vi "Grdifruit Fridge Control program with improved reading and logging (1).vi"() -> ()   [LabVIEW 2020]
uses:
  03e38eda-cf4e-4072-9910-2f004f8baa0f.vi
  <extravilib>/ChannelInstances/Tag-dbl/Write With Abort.vi
  <extravilib>/ChannelInstances/Tag-exp/Write With Abort.vi
  <extravilib>/ChannelInstances/Tag-dbl/Read With Abort.vi
  <extravilib>/ChannelInstances/Tag-exp/Read With Abort.vi
  <extravilib>/ChannelInstances/Tag-bool/Write With Abort.vi
  <extravilib>/ChannelInstances/Tag-bool/Read With Abort.vi
  <extravilib>/ChannelInstances/Tag-c(stamp,stamp,stamp,a[.](dbl),dbl)/Read With Abort.vi
  <extravilib>/ChannelInstances/Tag-c(stamp,stamp,stamp,a[.](dbl),dbl)/Write With Abort.vi
  <extravilib>/ChannelInstances/Tag-c(stamp,stamp,stamp,a[.](dbl),dbl)/Instantiate.vi
  <extravilib>/ChannelInstances/Tag-c(stamp,stamp,stamp,a[.](dbl),dbl)/Endpoint.vi
  <extravilib>/ChannelInstances/Tag-dbl/Instantiate.vi
  <extravilib>/ChannelInstances/Tag-bool/Instantiate.vi
  <extravilib>/ChannelInstances/Tag-exp/Instantiate.vi
  <extravilib>/ChannelInstances/Tag-c(stamp,stamp,stamp,a[.](dbl),dbl)/EndpointRead.vi
  <extravilib>/ChannelInstances/Tag-dbl/EndpointRead.vi
  <extravilib>/ChannelInstances/Tag-bool/EndpointRead.vi
  <extravilib>/ChannelInstances/Tag-exp/EndpointRead.vi
  <vilib>/Analysis/2dsp.llb/Upsample (DBL).vi
  <vilib>/express/express shared/transition.llb/Dynamic To Waveform Array.vi
  <vilib>/express/express signal manip/GetorSetDDTAttributes/Set DDT Attributes/SetT0.vi
  <vilib>/express/express shared/transition.llb/Waveform Array To Dynamic.vi
  <extravilib>/ChannelInstances/Tag-dbl/Endpoint.vi
  <extravilib>/ChannelInstances/Tag-exp/Endpoint.vi
  <extravilib>/ChannelInstances/Tag-bool/Endpoint.vi
  <vilib>/express/express signal manip/GetorSetDDTAttributes/Set DDT Attributes/Set DDT Properties.xnode
  <extravilib>/ChannelInstances/Tag-bool.lvlib
  <extravilib>/ChannelInstances/Tag-dbl.lvlib
  <extravilib>/ChannelInstances/Tag-c(stamp,stamp,stamp,a[.](dbl),dbl).lvlib
  <extravilib>/ChannelInstances/Tag-exp.lvlib
  <vilib>/ptbypt/NI_PtbyPt.lvlib
  <vilib>/Analysis/NI_AALPro.lvlib
panel:
  out "Temperatures (present)":dbl[](array[numeric])
  out "Temperatures (historic)":dynamicdata(graph)
  out "Parsing error":string
  out "raw XML":string
  out "error out":errorcluster
  out "error out 2":errorcluster
  out "error out 3":errorcluster
  in  "Tab Control":T1(tab)
  in  "Minutes to start pre-cooling before event starts":dbl
  in  "Low temp boundary":dbl=15.0
  in  "High temp boundary":dbl=25.0
  in  "Desired Temp":dbl=20.0
  in  "Sample rate (Hz)":dbl=0.2
  in  "Samples":dbl=1.0
  in  "Timeout (Sec)":dbl=10.0
  in  "Enable Logging 2":bool caption="Enable"
  out "Saving/Logging Data 2":bool caption="Saving Data"
  in  "Path to log file 2":path=path "C:/Users/vwilso17/Documents/Grad School/testlogging.xlsx"
  in  "Append to Current File 2":bool caption="Enable"
  out "End time":timestamp
  out "Start time":timestamp
  in  "Poll ADR signal":bool
  out "Price":dbl
  out "duration":dbl[](array[numeric])
  in  "ADR file path":path=path "C:/Users/vwilso17/Documents/Grad School/projects/Grid Fruit HVAC Project/CPPpayload.txt"
  out "Current time":timestamp
  in  "Stop communication with PI":bool
  out "Temp Above Limit":bool
  out "Temp Below Limit":bool
  out "Compressor on":bool
  out "ADR enabled":bool
  in  "Short Cycle wait time (ms)":dbl
  in  "Enable Short cycle protection":bool
  # "Evaporator Surface\n\nInterior Air \n\nInterior Surface\n\nExterior surface"
  # "Timeout>=samples/sample rate\n\nor \n\nsample rate>=samples/Timeout"
  # "Weeks\nDays\nHour\nMinutes\nSeconds"
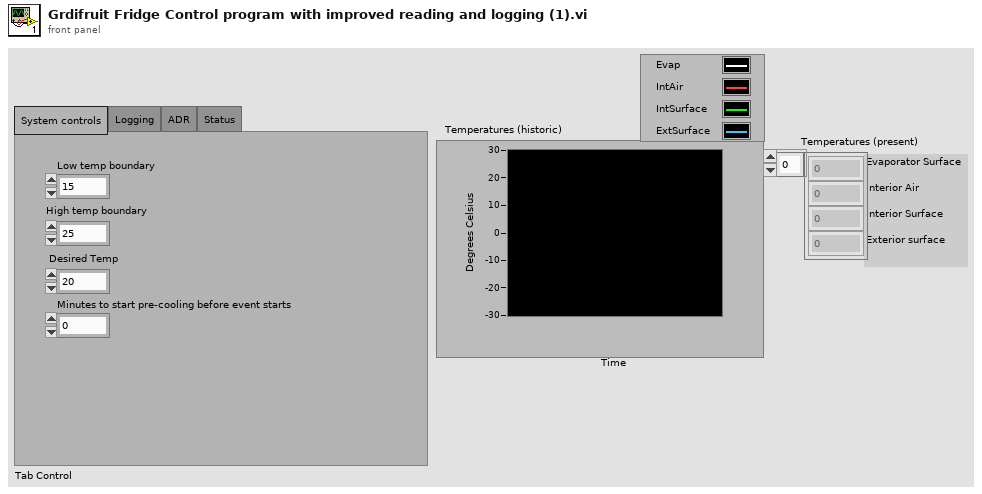
[diagram p1: front panel]
types:
  T1 = enum32{"System controls", "Logging", "ADR", "Status"}
  T2 = typedef "Tag-dbl.lvlib/))Channel.ctl" = refnum<queue>
  T3 = typedef "Tag-exp.lvlib/))Channel.ctl" = refnum<queue>
  T4 = cluster{"Current time":timestamp, "Start time":timestamp, "End time":timestamp, "duration":dbl[], "Price":dbl}
  T5 = cluster{"seconds since 1Jan1904":timestamp, "seconds since 1Jan1904":timestamp, "seconds since 1Jan1904":timestamp, "duration":dbl[], "Price":dbl}
  T6 = typedef "Tag-c(stamp,stamp,stamp,a[.](dbl),dbl).lvlib/))Channel.ctl" = refnum<queue>
  T7 = typedef "Tag-bool.lvlib/))Channel.ctl" = refnum<queue>
  T8 = enum16{"big-endian, network order", "native, host order", "little-endian"}
  T9 = cluster{"element":bool, "element":dbl, "element":dbl, "element":dbl, "element":dbl, "element":bool, timestamp, "Start time":timestamp, "End time":timestamp, "duration":dbl[], "Price":dbl, "element":dbl}
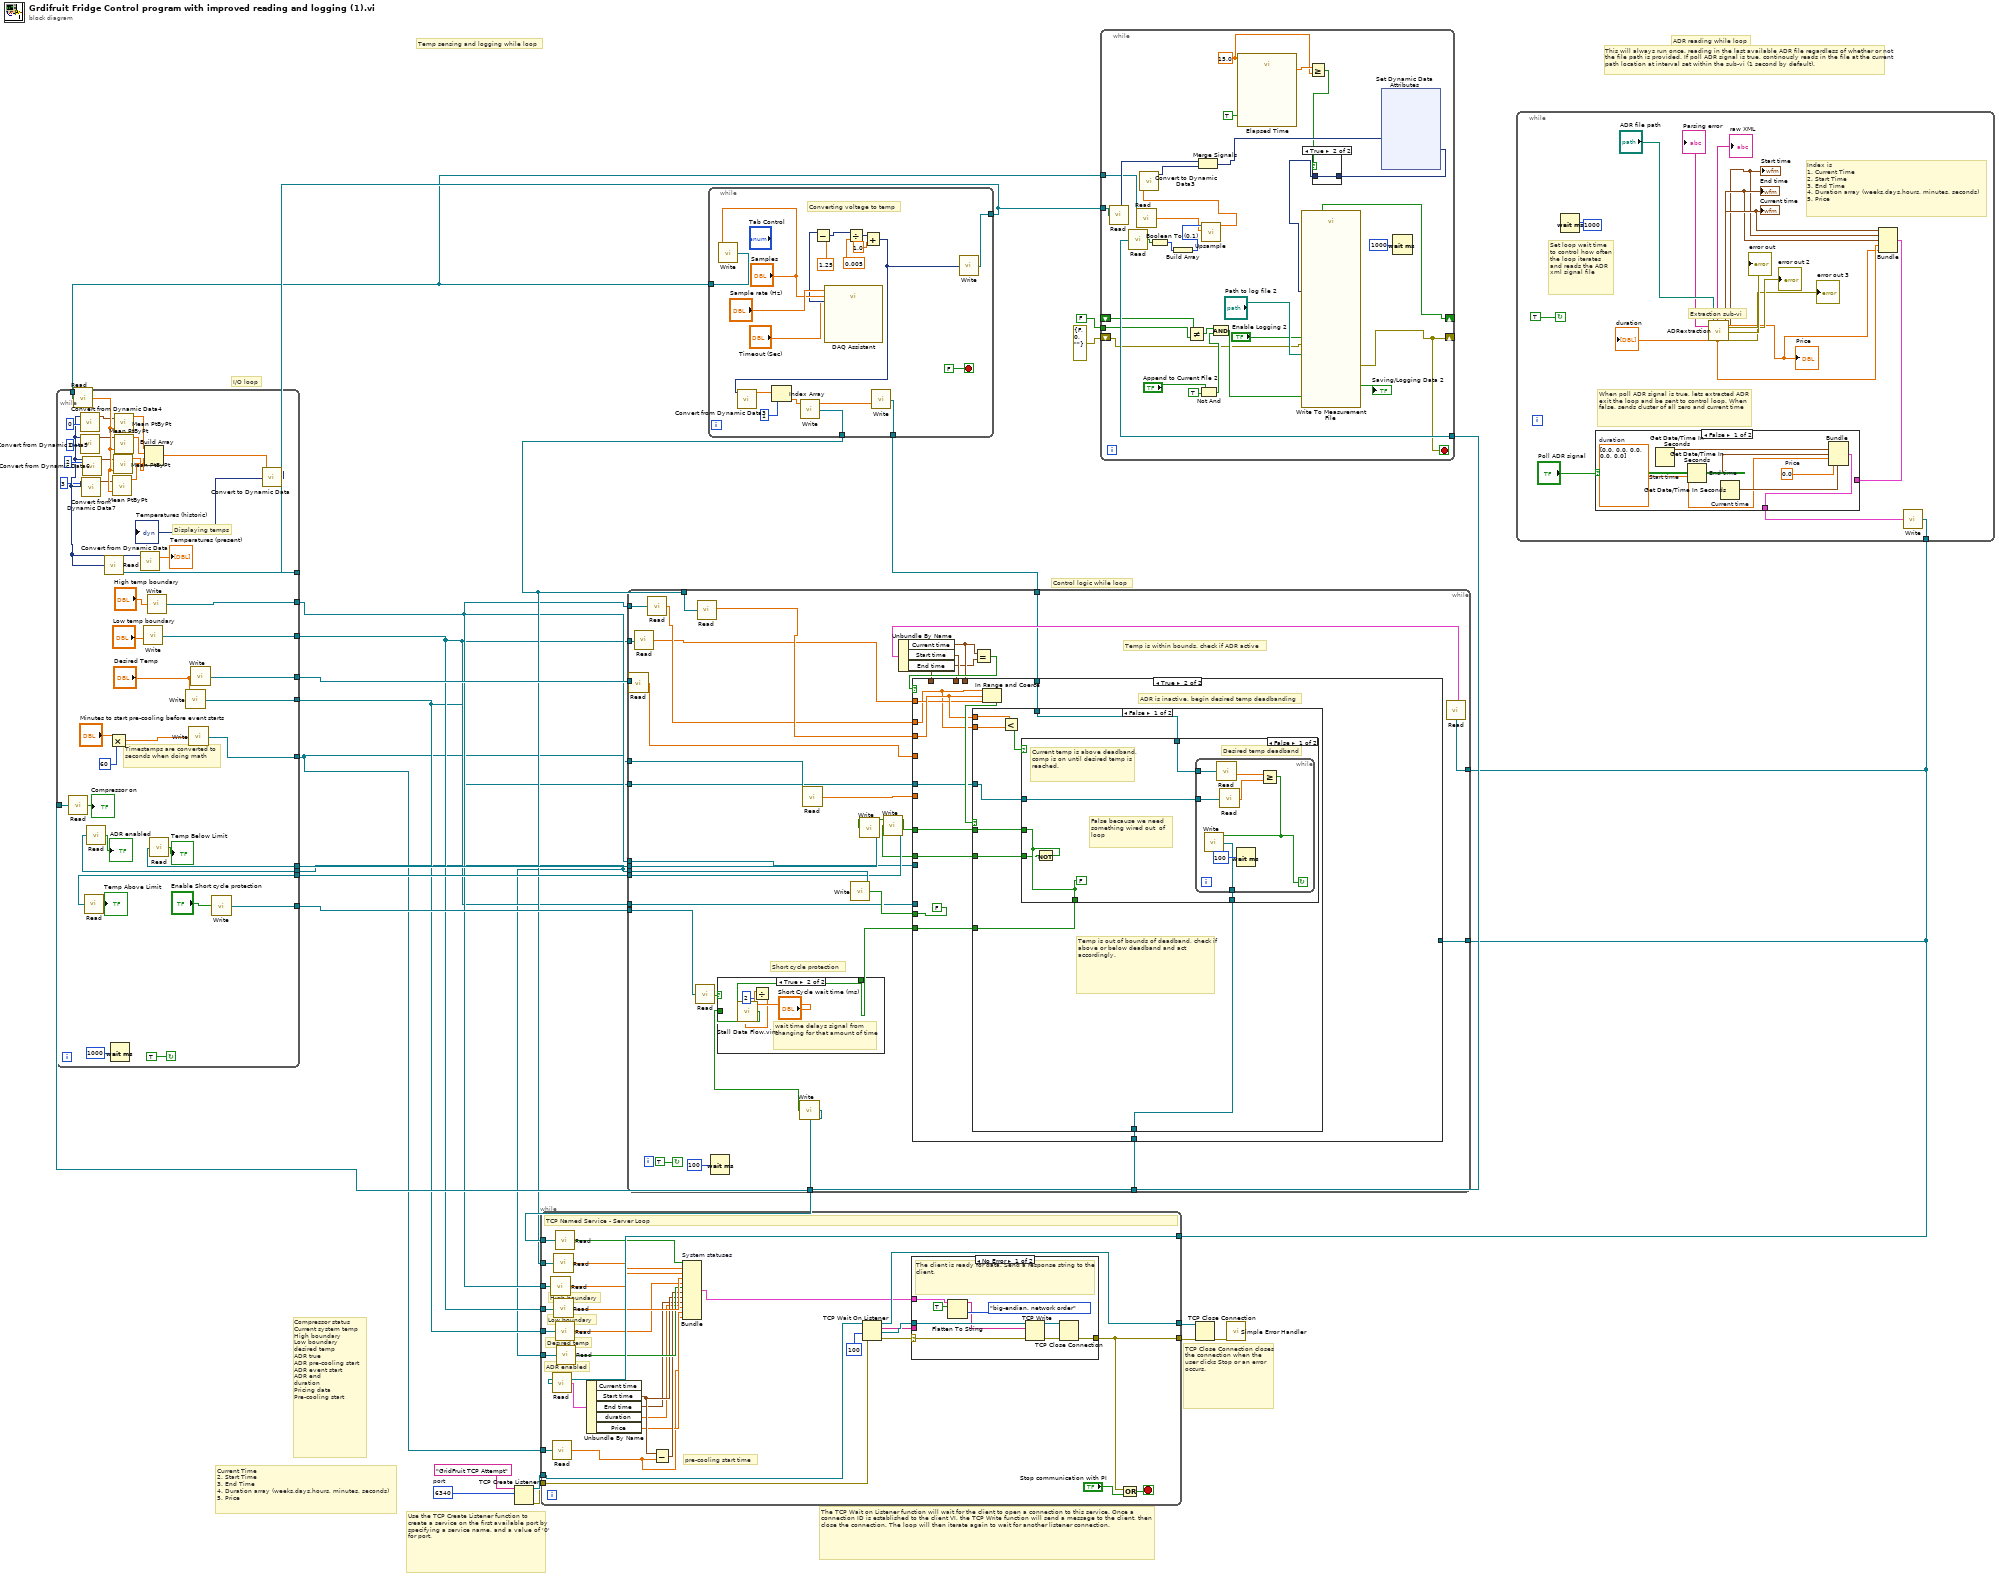
[diagram p0: block diagram]
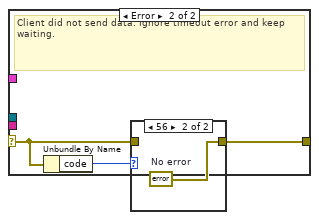
[diagram p3: hidden frame]
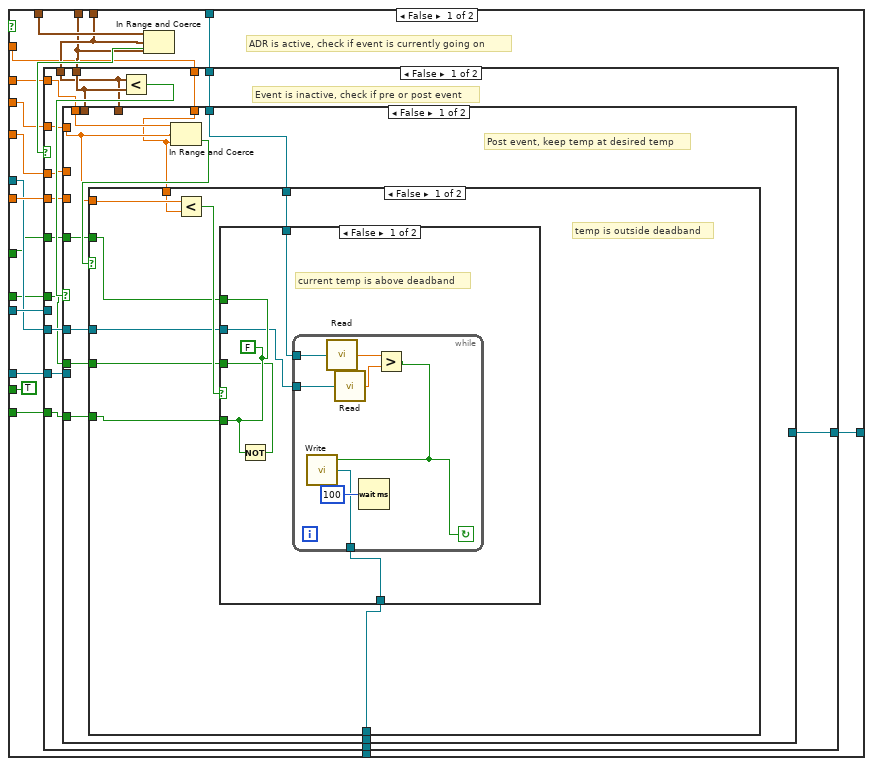
[diagram p5: hidden frame]
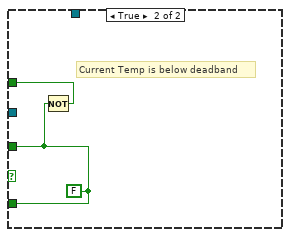
[diagram p6: hidden frame]
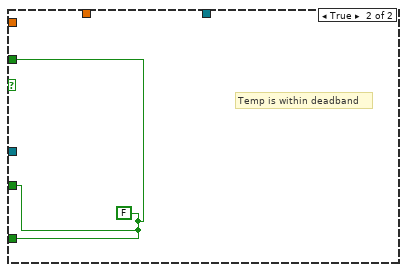
[diagram p7: hidden frame]
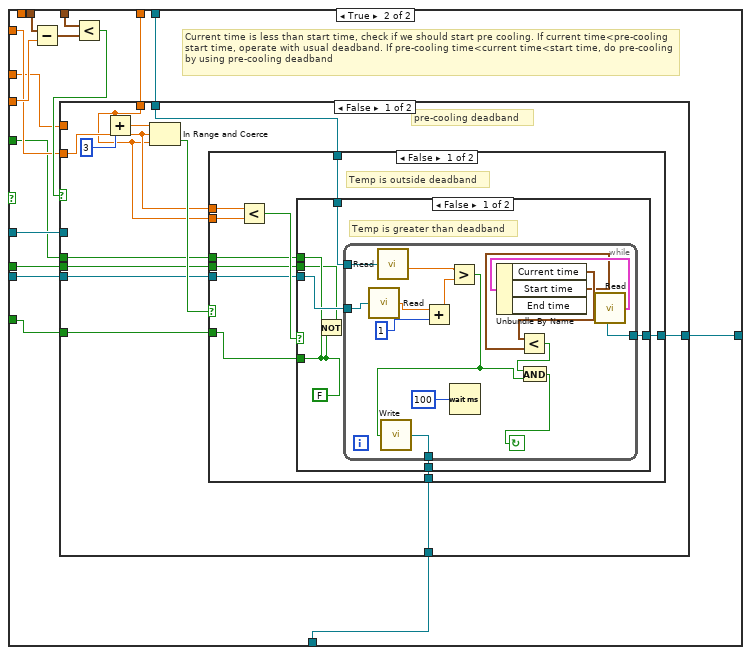
[diagram p8: hidden frame]
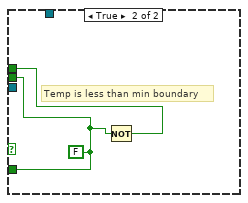
[diagram p9: hidden frame]
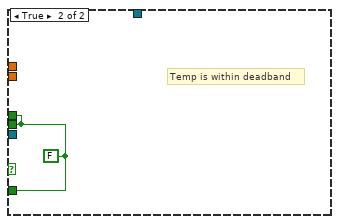
[diagram p10: hidden frame]
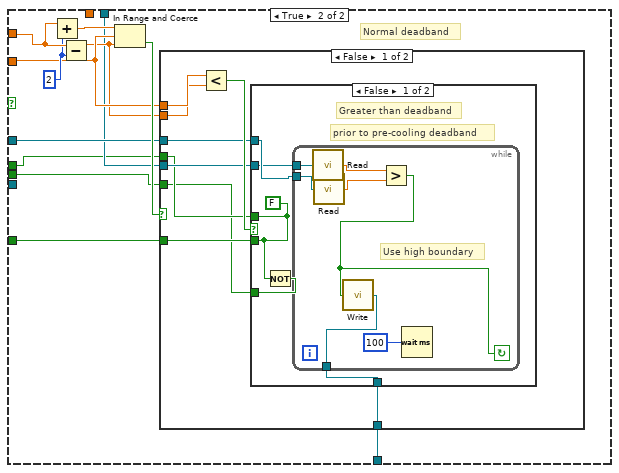
[diagram p11: hidden frame]
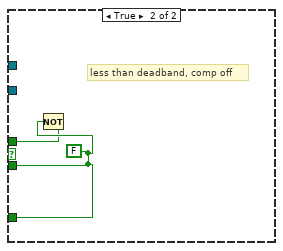
[diagram p12: hidden frame]
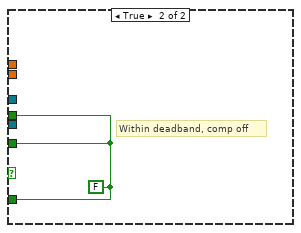
[diagram p13: hidden frame]
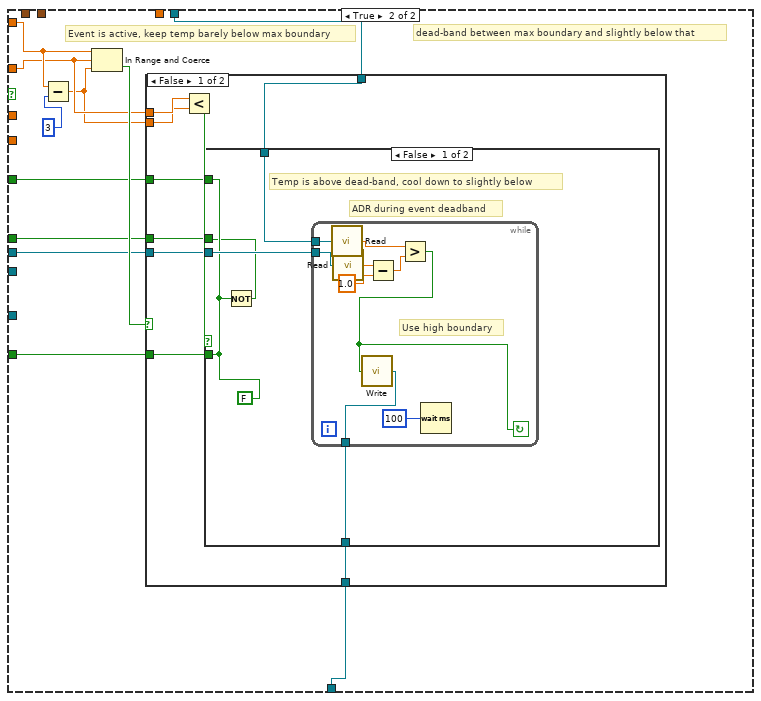
[diagram p14: hidden frame]
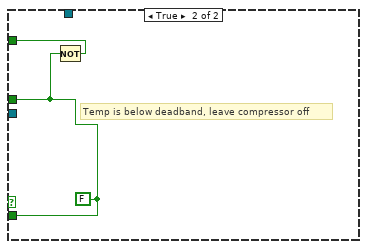
[diagram p15: hidden frame]
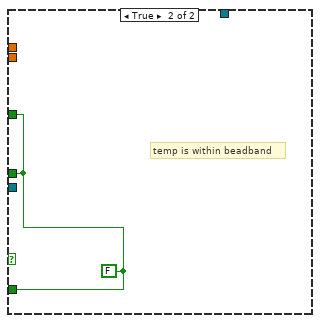
[diagram p16: hidden frame]
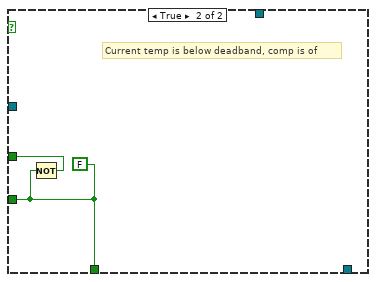
[diagram p17: hidden frame]
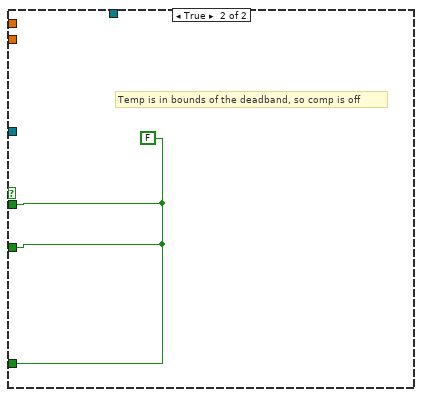
[diagram p18: hidden frame]
diagram:
  w19 = u16 6340  # port
  # "Current Time\n2. Start Time\n3. End Time\n4. Duration array (weeks,days,hours, minutes, seconds)\n5. Price"
  # "Compressor status\nCurrent system temp\nHigh boundary\nLow boundary\ndesired temp\nADR true\nADR pre-cooling start\nADR event start\nADR end\nduration\nPricing data\nPre-cooling start"
  # "I/O loop"
  # "TCP Close Connection closes the connection when the user clicks Stop or an error occurs."
  # "The TCP Wait on Listener function will wait for the client to open a connection to this service. Once a connection ID is established to the client VI, the TCP Write function will send a message to the client, then close the connection. The loop will then iterate again to wait for another listener connection."
  # "Use the TCP Create Listener function to create a service on the first available port by specifying a service name, and a value of '0' for port."
  # "Control logic while loop"
  # "Temp sensing and logging while loop"
  # "This will always run once, reading in the last available ADR file regardless of whether or not the file path is provided. If poll ADR signal is true, continously reads in the file at the current path location at interval set within the sub-vi (1 second by default)."
  # "ADR reading while loop"
  n1 = TCP Create Listener(10:w19, 11:"GridFruit TCP Attempt" ("service name")) -> (0:w23:errorcluster, 3:w24:refnum<k5>)  [unwired: 3 in, 1 out]
  n2 = while {
    tunnel: [w32] -> w7
    tunnel: [w31] -> w14
    tunnel: [w26] -> w9
    tunnel: [w25] -> w8
    stop <- FALSE stop-if-true
    # "Converting voltage to temp"
    n3 = call <extravilib>:"Write.vi"("element"="Samples") -> ("channel"=w25:T2)  [unwired: 1 out]
    n4 = call "DAQ Assistant"("rate"="Sample rate (Hz)", "number of samples"="Samples", "timeout (s)"="Timeout (Sec)") -> ("data"=w37:dynamicdata)  [unwired: 13 in, 3 out]
    n5 = Subtract(x=w37, y=1.25) -> (x-y=w40:dynamicdata)
    n6 = Divide(x=w40, y=0.005) -> (x/y=w30:dynamicdata)
    n7 = Add(x=w30, y=1.0) -> (x+y=w27:dynamicdata)
    n8 = call "Convert from Dynamic Data3"("Dynamic Data Type"=w27) -> ("Array"=w35:dbl[])  [unwired: 3 in]
    n9 = Index Array(array=w35, index=1) -> (element=w33:dbl)
    n10 = call <extravilib>:"Write.vi"("element"=w33) -> ("channel"=w32:T2)  [unwired: 1 out]
    n11 = call <extravilib>:"Write.vi"("element"=w33) -> ("channel"=w31:T2)  [unwired: 1 out]
    n12 = call <extravilib>:"Write.vi"("element"=w27) -> ("channel"=w26:T3)  [unwired: 1 out]
  }
  n13 = while {
    tunnel: [w44] -> w1
    stop <- TRUE continue-if-true
    # "Index is\n1. Current Time\n2. Start Time\n3. End Time\n4. Duration array (weeks,days,hours, minutes, seconds)\n5. Price"
    # "Set loop wait time to control how often the loop iterates and reads the ADR xml signal file"
    # "When poll ADR signal is true, lets extracted ADR exit the loop and be sent to control loop. When false, sends cluster of all zero and current time"
    # "Extraction sub-vi"
    n14 = Wait (ms)(milliseconds to wait=1000) -> ()  [unwired: 1 out]
    n15 = call "ADRextraction.vi"("Path in"="ADR file path") -> ("Error"=→"Parsing error":string, "raw xML"=→"raw XML":string, "duration"=w46:dbl[], "Start time"=w43:timestamp, "End time"=w51:timestamp, "Current time"=w52:timestamp, "Price"=w45:dbl, "error out 2"=→"error out 2":errorcluster, 24:"error out"=→"error out":errorcluster, 27:"error out"=→"error out 3":errorcluster)  [unwired: 12 in, 5 out]
    "Price" <- w45
    "duration" <- w46
    "Start time" <- w43
    "End time" <- w51
    "Current time" <- w52
    n16 = Bundle("Current time"=w52, "Start time"=w43, "End time"=w51, "duration"=w46, "Price"=w45) -> (w47:T4)  [unwired: 1 in]
    n17 = case shown="False" "Poll ADR signal" {
      tunnel: [w61 w66] -> w48
      tunnel: w47 -> [_ w66]
      frame False {
        w60 = dbl[] [0.0, 0.0, 0.0, 0.0, 0.0]  # duration
        w62 = 0.0  # Price
        n18 = Get Date/Time In Seconds "Start time"() -> (seconds since 1Jan1904=w63:timestamp)
        n19 = Get Date/Time In Seconds "End time"() -> (seconds since 1Jan1904=w64:timestamp)
        n20 = Get Date/Time In Seconds "Current time"() -> (seconds since 1Jan1904=w65:timestamp)
        n21 = Bundle("seconds since 1Jan1904"=w65, "seconds since 1Jan1904"=w63, "seconds since 1Jan1904"=w64, "duration"=w60, "Price"=w62) -> (w61:T5)  [unwired: 1 in]
      }
      frame True {
      }
    }
    n22 = call <extravilib>:"Write.vi"("element"=w48) -> ("channel"=w44:T6)  [unwired: 1 out]
  }
  n23 = while {
    tunnel: [w106] -> w6
    tunnel: [w104] -> w5
    tunnel: [w102] -> w18
    tunnel: [w98] -> w2
    tunnel: w12 -> [w96]
    tunnel: w3 -> [w94]
    tunnel: w17 -> [w92]
    tunnel: w16 -> [w90]
    tunnel: [w87] -> w15
    tunnel: [w86] -> w4
    tunnel: w9 -> [w85]
    tunnel: w8 -> [w81]
    stop <- TRUE continue-if-true
    # "Displaying temps"
    # "Timestamps are converted to seconds when doing math"
    n24 = call <extravilib>:"Read.vi"("channel"=w96) -> ("element"=→"Compressor on":bool)  [unwired: 1 in, 1 out]
    n25 = call <extravilib>:"Read.vi"("channel"=w81) -> ("element"=w77:dbl)  [unwired: 1 in, 1 out]
    n26 = call <extravilib>:"Read.vi"("channel"=w90) -> ("element"=→"Temp Above Limit":bool)  [unwired: 1 in, 1 out]
    n27 = call <extravilib>:"Read.vi"("channel"=w94) -> ("element"=→"ADR enabled":bool)  [unwired: 1 in, 1 out]
    n28 = call <extravilib>:"Read.vi"("channel"=w85) -> ("element"=w71:dynamicdata)  [unwired: 1 in, 1 out]
    n29 = call "Convert from Dynamic Data4"("Dynamic Data Type"=w71, "Channel"=0) -> ("Waveform"=w76:waveform(dbl))  [unwired: 2 in]
    n30 = call "Convert from Dynamic Data5"("Dynamic Data Type"=w71, "Channel"=1) -> ("Waveform"=w75:waveform(dbl))  [unwired: 2 in]
    n31 = call "Convert from Dynamic Data7"("Dynamic Data Type"=w71, "Channel"=3) -> ("Waveform"=w70:waveform(dbl))  [unwired: 2 in]
    n32 = call "Convert from Dynamic Data6"("Dynamic Data Type"=w71, "Channel"=2) -> ("Waveform"=w73:waveform(dbl))  [unwired: 2 in]
    n33 = Multiply(x="Minutes to start pre-cooling before event starts", y=60) -> (x*y=w99:dbl)
    n34 = Wait (ms)(milliseconds to wait=u32 1000) -> ()  [unwired: 1 out]
    n35 = call <vilib>:"Mean PtByPt.vi"("x"=w70, "sample length"=w77) -> ("mean"=w78:dbl)  [unwired: 2 in, 1 out]
    n36 = call <vilib>:"Mean PtByPt.vi"("x"=w73, "sample length"=w77) -> ("mean"=w79:dbl)  [unwired: 2 in, 1 out]
    n37 = call <vilib>:"Mean PtByPt.vi"("x"=w76, "sample length"=w77) -> ("mean"=w84:dbl)  [unwired: 2 in, 1 out]
    n38 = call <vilib>:"Mean PtByPt.vi"("x"=w75, "sample length"=w77) -> ("mean"=w80:dbl)  [unwired: 2 in, 1 out]
    n39 = call "Convert from Dynamic Data"("Dynamic Data Type"=w71) -> ("Array"=→"Temperatures (present)":dbl[])  [unwired: 3 in]
    n40 = call <extravilib>:"Write.vi"("element"="Low temp boundary") -> ("channel"=w104:T2)  [unwired: 1 out]
    n41 = Build Array(w84, w80, w79, w78) -> (w83:dbl[])
    n42 = call <extravilib>:"Write.vi"("element"="High temp boundary") -> ("channel"=w106:T2)  [unwired: 1 out]
    n43 = call <extravilib>:"Read.vi"("channel"=w92) -> ("element"=→"Temp Below Limit":bool)  [unwired: 1 in, 1 out]
    n44 = call <extravilib>:"Write.vi"("element"="Desired Temp") -> ("channel"=w86:T2)  [unwired: 1 out]
    n45 = call <extravilib>:"Write.vi"("element"=w99) -> ("channel"=w98:T2)  [unwired: 1 out]
    n46 = call <extravilib>:"Write.vi"("element"="Desired Temp") -> ("channel"=w102:T2)  [unwired: 1 out]
    n47 = call <extravilib>:"Write.vi"("element"="Enable Short cycle protection") -> ("channel"=w87:T7)  [unwired: 1 out]
    n48 = call "Convert to Dynamic Data"("Array"=w83) -> ("Dynamic Data Type"=→"Temperatures (historic)":dynamicdata)  [unwired: 3 in]
  }
  n49 = while {
    tunnel: w1 -> [w140]
    tunnel: w7 -> [w137]
    tunnel: w6 -> [w135]
    tunnel: w5 -> [w133]
    tunnel: w18 -> [w131]
    tunnel: w2 -> [w129]
    tunnel: [w127] -> w12
    tunnel: [w125] -> w3
    tunnel: [w124] -> w17
    tunnel: [w123] -> w16
    tunnel: w15 -> [w122]
    tunnel: w4 -> [w120]
    tunnel: w14 -> [w119]
    tunnel: w12 -> [w118]
    tunnel: w6 -> [w117]
    tunnel: w5 -> [w116]
    tunnel: w1 -> [w109]
    stop <- TRUE continue-if-true
    # "Temp is within bounds, check if ADR active"
    # "Short cycle protection"
    n50 = call <extravilib>:"Read.vi"("channel"=w131) -> ("element"=w130:dbl)  [unwired: 1 in, 1 out]
    n51 = call <extravilib>:"Read.vi"("channel"=w133) -> ("element"=w132:dbl)  [unwired: 1 in, 1 out]
    n52 = call <extravilib>:"Read.vi"("channel"=w135) -> ("element"=w134:dbl)  [unwired: 1 in, 1 out]
    n53 = call <extravilib>:"Read.vi"("channel"=w122) -> ("element"=w121:bool)  [unwired: 1 in, 1 out]
    n54 = call <extravilib>:"Read.vi"("channel"=w137) -> ("element"=w136:dbl)  [unwired: 1 in, 1 out]
    n55 = Wait (ms)(milliseconds to wait=u32 100) -> ()  [unwired: 1 out]
    n56 = call <extravilib>:"Read.vi"("channel"=w129) -> ("element"=w128:dbl)  [unwired: 1 in, 1 out]
    n57 = call <extravilib>:"Read.vi"("channel"=w140) -> ("element"=w139:T4)  [unwired: 1 in, 1 out]
    n58 = Unbundle By Name(w139) -> ("Current time"=w114:timestamp, "Start time"=w113:timestamp, "End time"=w112:timestamp)
    n59 = Equal?(x=w114, y=w112) -> (x = y?=w115:bool)
    n60 = case shown="True" w115 {
      tunnel: w136 -> [w157 w355]
      tunnel: w130 -> [w156 _]
      tunnel: [w155 w357] -> w143
      tunnel: [TRUE FALSE] -> w126
      tunnel: w114 -> [w159 _]
      tunnel: w113 -> [w158 _]
      tunnel: w112 -> [w161 _]
      tunnel: w134 -> [w154 w348]
      tunnel: w128 -> [w153 _]
      tunnel: w132 -> [w152 w349]
      tunnel: w120 -> [w147 w354]
      tunnel: w119 -> [w150 w353]
      tunnel: [w149 w352] -> w118
      tunnel: w117 -> [w151 _]
      tunnel: w116 -> [w148 _]
      tunnel: [w146 w351] -> w111
      tunnel: [w145 w350] -> w110
      tunnel: w109 -> [w144 _]
      frame False {
        # "ADR is active, check if event is currently going on"
        n61 = In Range and Coerce(upper limit=w161, x=w159, lower limit=w158) -> (In Range?=w160:bool)  [unwired: 1 out]
        n62 = case shown="False" w160 {
          tunnel: w159 -> [w172 _]
          tunnel: w158 -> [w173 _]
          tunnel: w157 -> [w177 w317]
          tunnel: w156 -> [w176 _]
          tunnel: [w175 w318] -> w155
          tunnel: w154 -> [w163 w321]
          tunnel: w153 -> [w174 _]
          tunnel: w152 -> [w171 _]
          tunnel: w151 -> [_ w315]
          tunnel: w150 -> [w170 w314]
          tunnel: [w169 w313] -> w149
          tunnel: w148 -> [w168 _]
          tunnel: w147 -> [w167 _]
          tunnel: [w166 w312] -> w146
          tunnel: [w165 w311] -> w145
          tunnel: w144 -> [w164 _]
          frame False {
            # "Event is inactive, check if pre or post event"
            n63 = Less?(x=w172, y=w173) -> (x < y?=w178:bool)
            n64 = case shown="False" w178 {
              tunnel: w177 -> [w186 w223]
              tunnel: w176 -> [_ w222]
              tunnel: [w187 w221] -> w175
              tunnel: w174 -> [_ w228]
              tunnel: w173 -> [_ w227]
              tunnel: w172 -> [_ w226]
              tunnel: w171 -> [w180 w220]
              tunnel: w170 -> [w185 w218]
              tunnel: [w184 w219] -> w169
              tunnel: w168 -> [_ w217]
              tunnel: w167 -> [w179 w216]
              tunnel: [w183 w215] -> w166
              tunnel: [w182 w214] -> w165
              tunnel: w164 -> [_ w213]
              tunnel: w163 -> [w181 _]
              frame False {
                # "Post event, keep temp at desired temp"
                n65 = In Range and Coerce(upper limit=w181, x=w186, lower limit=w180) -> (In Range?=w188:bool)  [unwired: 1 out]
                n66 = case shown="False" w188 {
                  tunnel: [w195 w212] -> w187
                  tunnel: w186 -> [w197 _]
                  tunnel: w185 -> [w194 _]
                  tunnel: [w193 _] -> w184
                  tunnel: [w192 w212] -> w183
                  tunnel: [w191 w212] -> w182
                  tunnel: w180 -> [w190 _]
                  tunnel: w179 -> [w189 _]
                  frame False {
                    # "temp is outside deadband"
                    n67 = Less?(x=w197, y=w190) -> (x < y?=w196:bool)
                    n68 = case shown="False" w196 {
                      tunnel: [w200 w211] -> w195
                      tunnel: w194 -> [w202 _]
                      tunnel: [w201 _] -> w193
                      tunnel: [w199 w211] -> w192
                      tunnel: [w200 w210] -> w191
                      tunnel: w189 -> [w198 _]
                      frame False {
                        w200 = FALSE
                        # "current temp is above deadband"
                        n69 = Not(x=w200) -> (.not. x?=w199:bool)
                        n70 = while {
                          tunnel: w202 -> [w208]
                          tunnel: [w207] -> w201
                          tunnel: w198 -> [w204]
                          stop <- w205 continue-if-true
                          n71 = call <extravilib>:"Read.vi"("channel"=w208) -> ("element"=w206:dbl)  [unwired: 1 in, 1 out]
                          n72 = call <extravilib>:"Read.vi"("channel"=w204) -> ("element"=w203:dbl)  [unwired: 1 in, 1 out]
                          n73 = Wait (ms)(milliseconds to wait=u32 100) -> ()  [unwired: 1 out]
                          n74 = Greater?(x=w206, y=w203) -> (0:w205:bool)
                          n75 = call <extravilib>:"Write.vi"("element"=w205) -> ("channel"=w207:T7)  [unwired: 1 out]
                        }
                      }
                      frame True {
                        w211 = FALSE
                        # "Current Temp is below deadband"
                        n76 = Not(x=w211) -> (.not. x?=w210:bool)
                      }
                    }
                  }
                  frame True {
                    w212 = FALSE
                    # "Temp is within deadband"
                  }
                }
              }
              frame True {
                # "Current time is less than start time, check if we should start pre cooling. If current time<pre-cooling start time, operate with usual deadband. If pre-cooling time<current time<start time, do pre-cooling by using pre-cooling deadband"
                n77 = Subtract(x=w227, y=w228) -> (x-y=w225:timestamp)
                n78 = Less?(x=w226, y=w225) -> (x < y?=w224:bool)
                n79 = case shown="False" w224 {
                  tunnel: w223 -> [w237 w281]
                  tunnel: w222 -> [_ w285]
                  tunnel: [w235 w282] -> w221
                  tunnel: w220 -> [w236 _]
                  tunnel: [w234 w277] -> w219
                  tunnel: w218 -> [w233 w278]
                  tunnel: w217 -> [w232 _]
                  tunnel: w216 -> [_ w279]
                  tunnel: [w231 w276] -> w215
                  tunnel: [w230 w275] -> w214
                  tunnel: w213 -> [w229 _]
                  frame False {
                    # "pre-cooling deadband"
                    n80 = Add(x=w236, y=3) -> (x+y=w239:dbl)
                    n81 = In Range and Coerce(upper limit=w239, x=w237, lower limit=w236) -> (In Range?=w238:bool)  [unwired: 1 out]
                    n82 = case shown="False" w238 {
                      tunnel: w237 -> [w248 _]
                      tunnel: w236 -> [w247 _]
                      tunnel: [w249 w274] -> w235
                      tunnel: [w246 _] -> w234
                      tunnel: w233 -> [w245 _]
                      tunnel: w232 -> [w244 _]
                      tunnel: [w242 w274] -> w231
                      tunnel: [w243 w274] -> w230
                      tunnel: w229 -> [w241 _]
                      frame False {
                        # "Temp is outside deadband"
                        n83 = Less?(x=w248, y=w247) -> (x < y?=w250:bool)
                        n84 = case shown="False" w250 {
                          tunnel: [w253 w273] -> w249
                          tunnel: [w256 _] -> w246
                          tunnel: w245 -> [w255 _]
                          tunnel: w244 -> [w254 _]
                          tunnel: [w253 w272] -> w243
                          tunnel: [w252 w273] -> w242
                          tunnel: w241 -> [w251 _]
                          frame False {
                            w253 = FALSE
                            # "Temp is greater than deadband"
                            n85 = Not(x=w253) -> (.not. x?=w252:bool)
                            n86 = while {
                              tunnel: w254 -> [w270]
                              tunnel: w255 -> [w269]
                              tunnel: [w268] -> w256
                              tunnel: w251 -> [w263]
                              stop <- w261 continue-if-true
                              n87 = call <extravilib>:"Read.vi"("channel"=w270) -> ("element"=w266:dbl)  [unwired: 1 in, 1 out]
                              n88 = call <extravilib>:"Read.vi"("channel"=w269) -> ("element"=w264:dbl)  [unwired: 1 in, 1 out]
                              n89 = Add(x=w266, y=1) -> (x+y=w265:dbl)
                              n90 = Greater?(x=w264, y=w265) -> (0:w260:bool)
                              n91 = call <extravilib>:"Write.vi"("element"=w260) -> ("channel"=w268:T7)  [unwired: 1 out]
                              n92 = Wait (ms)(milliseconds to wait=u32 100) -> ()  [unwired: 1 out]
                              n93 = call <extravilib>:"Read.vi"("channel"=w263) -> ("element"=w262:T4)  [unwired: 1 in, 1 out]
                              n94 = Unbundle By Name(w262) -> ("Current time"=w259:timestamp, "Start time"=w258:timestamp)  [unwired: 1 out]
                              n95 = Less?(x=w259, y=w258) -> (x < y?=w257:bool)
                              n96 = And(x=w257, y=w260) -> (x .and. y?=w261:bool)
                            }
                          }
                          frame True {
                            w273 = FALSE
                            # "Temp is less than min boundary"
                            n97 = Not(x=w273) -> (.not. x?=w272:bool)
                          }
                        }
                      }
                      frame True {
                        w274 = FALSE
                        # "Temp is within deadband"
                      }
                    }
                  }
                  frame True {
                    w284 = 2
                    # "Normal deadband"
                    n98 = Add(x=w285, y=w284) -> (x+y=w286:dbl)
                    n99 = Subtract(x=w285, y=w284) -> (x-y=w280:dbl)
                    n100 = In Range and Coerce(upper limit=w286, x=w281, lower limit=w280) -> (In Range?=w283:bool)  [unwired: 1 out]
                    n101 = case shown="False" w283 {
                      tunnel: [w292 w310] -> w282
                      tunnel: w281 -> [w295 _]
                      tunnel: w280 -> [w294 _]
                      tunnel: w279 -> [w291 _]
                      tunnel: w278 -> [w290 _]
                      tunnel: [w289 _] -> w277
                      tunnel: [w287 w310] -> w276
                      tunnel: [w288 w310] -> w275
                      frame False {
                        n102 = Less?(x=w295, y=w294) -> (x < y?=w293:bool)
                        n103 = case shown="False" w293 {
                          tunnel: [w297 w309] -> w292
                          tunnel: w291 -> [w300 _]
                          tunnel: w290 -> [w299 _]
                          tunnel: [w298 _] -> w289
                          tunnel: [w297 w308] -> w288
                          tunnel: [w296 w309] -> w287
                          frame False {
                            w297 = FALSE
                            # "prior to pre-cooling deadband"
                            # "Greater than deadband"
                            n104 = Not(x=w297) -> (.not. x?=w296:bool)
                            n105 = while {
                              tunnel: [w305] -> w298
                              tunnel: w300 -> [w303]
                              tunnel: w299 -> [w302]
                              stop <- w304 continue-if-true
                              # "Use high boundary"
                              n106 = call <extravilib>:"Read.vi"("channel"=w302) -> ("element"=w306:dbl)  [unwired: 1 in, 1 out]
                              n107 = call <extravilib>:"Read.vi"("channel"=w303) -> ("element"=w301:dbl)  [unwired: 1 in, 1 out]
                              n108 = Greater?(x=w306, y=w301) -> (0:w304:bool)
                              n109 = call <extravilib>:"Write.vi"("element"=w304) -> ("channel"=w305:T7)  [unwired: 1 out]
                              n110 = Wait (ms)(milliseconds to wait=u32 100) -> ()  [unwired: 1 out]
                            }
                          }
                          frame True {
                            w309 = FALSE
                            # "less than deadband, comp off"
                            n111 = Not(x=w309) -> (.not. x?=w308:bool)
                          }
                        }
                      }
                      frame True {
                        w310 = FALSE
                        # "Within deadband, comp off"
                      }
                    }
                  }
                }
              }
            }
          }
          frame True {
            # "dead-band between max boundary and slightly below that"
            # "Event is active, keep temp barely below max boundary"
            n112 = Subtract(x=w321, y=3) -> (x-y=w316:dbl)
            n113 = In Range and Coerce(upper limit=w321, x=w317, lower limit=w316) -> (In Range?=w319:bool)  [unwired: 1 out]
            n114 = case shown="False" w319 {
              tunnel: [w327 w347] -> w318
              tunnel: w317 -> [w330 _]
              tunnel: w316 -> [w329 _]
              tunnel: [w326 _] -> w313
              tunnel: w315 -> [w325 _]
              tunnel: w314 -> [w324 _]
              tunnel: [w323 w347] -> w312
              tunnel: [w322 w347] -> w311
              frame False {
                n115 = Less?(x=w330, y=w329) -> (x < y?=w328:bool)
                n116 = case shown="False" w328 {
                  tunnel: [w332 w346] -> w327
                  tunnel: [w335 _] -> w326
                  tunnel: w325 -> [w334 _]
                  tunnel: w324 -> [w333 _]
                  tunnel: [w331 w346] -> w323
                  tunnel: [w332 w345] -> w322
                  frame False {
                    w332 = FALSE
                    # "ADR during event deadband"
                    # "Temp is above dead-band, cool down to slightly below"
                    n117 = Not(x=w332) -> (.not. x?=w331:bool)
                    n118 = while {
                      tunnel: [w339] -> w335
                      tunnel: w334 -> [w337]
                      tunnel: w333 -> [w336]
                      stop <- w338 continue-if-true
                      # "Use high boundary"
                      n119 = call <extravilib>:"Read.vi"("channel"=w336) -> ("element"=w341:dbl)  [unwired: 1 in, 1 out]
                      n120 = call <extravilib>:"Read.vi"("channel"=w337) -> ("element"=w343:dbl)  [unwired: 1 in, 1 out]
                      n121 = Subtract(x=w343, y=1.0) -> (x-y=w340:dbl)
                      n122 = Greater?(x=w341, y=w340) -> (0:w338:bool)
                      n123 = call <extravilib>:"Write.vi"("element"=w338) -> ("channel"=w339:T7)  [unwired: 1 out]
                      n124 = Wait (ms)(milliseconds to wait=u32 100) -> ()  [unwired: 1 out]
                    }
                  }
                  frame True {
                    w346 = FALSE
                    # "Temp is below deadband, leave compressor off"
                    n125 = Not(x=w346) -> (.not. x?=w345:bool)
                  }
                }
              }
              frame True {
                w347 = FALSE
                # "temp is within beadband"
              }
            }
          }
        }
      }
      frame True {
        # "ADR is inactive, begin desired temp deadbanding"
        n126 = In Range and Coerce(upper limit=w348, x=w355, lower limit=w349) -> (In Range?=w358:bool)  [unwired: 1 out]
        n127 = case shown="False" w358 {
          tunnel: [w365 w382] -> w357
          tunnel: w355 -> [w367 _]
          tunnel: w354 -> [w364 _]
          tunnel: w353 -> [w363 _]
          tunnel: [w362 _] -> w352
          tunnel: [w361 w382] -> w351
          tunnel: [w360 w382] -> w350
          tunnel: w348 -> [w359 _]
          frame False {
            # "Temp is out of bounds of deadband, check if above or below deadband and act accordingly."
            n128 = Less?(x=w367, y=w359) -> (x < y?=w366:bool)
            n129 = case shown="False" w366 {
              tunnel: [w369 w381] -> w365
              tunnel: w364 -> [w372 _]
              tunnel: w363 -> [w371 _]
              tunnel: [w370 _] -> w362
              tunnel: [w368 w381] -> w361
              tunnel: [w369 w380] -> w360
              frame False {
                w369 = FALSE
                # "Desired temp deadband"
                # "False because we need something wired out  of loop"
                # "Current temp is above deadband, comp is on until desired temp is reached."
                n130 = Not(x=w369) -> (.not. x?=w368:bool)
                n131 = while {
                  tunnel: w372 -> [w377]
                  tunnel: w371 -> [w375]
                  tunnel: [w374] -> w370
                  stop <- w373 continue-if-true
                  n132 = call <extravilib>:"Read.vi"("channel"=w375) -> ("element"=w378:dbl)  [unwired: 1 in, 1 out]
                  n133 = call <extravilib>:"Read.vi"("channel"=w377) -> ("element"=w376:dbl)  [unwired: 1 in, 1 out]
                  n134 = Wait (ms)(milliseconds to wait=u32 100) -> ()  [unwired: 1 out]
                  n135 = Greater Or Equal?(x=w378, y=w376) -> (x >= y?=w373:bool)
                  n136 = call <extravilib>:"Write.vi"("element"=w373) -> ("channel"=w374:T7)  [unwired: 1 out]
                }
              }
              frame True {
                w381 = FALSE
                # "Current temp is below deadband, comp is of"
                n137 = Not(x=w381) -> (.not. x?=w380:bool)
              }
            }
          }
          frame True {
            w382 = FALSE
            # "Temp is in bounds of the deadband, so comp is off"
          }
        }
      }
    }
    n138 = case shown="True" w121 {
      tunnel: [w383 w387] -> w138
      tunnel: w143 -> [w383 w388]
      frame False {
      }
      frame True {
        # "wait time delays signal from changing for that amount of time"
        n139 = Divide(x="Short Cycle wait time (ms)", y=2) -> (x/y=w384:dbl)
        n140 = call "Stall Data Flow.vim"("value in"=w388, "milliseconds to wait"=w384) -> ("value out"=w387:bool)  [unwired: 1 out]
      }
    }
    n141 = call <extravilib>:"Write.vi"("element"=w138) -> ("channel"=w127:T7)  [unwired: 1 out]
    n142 = call <extravilib>:"Write.vi"("element"=w126) -> ("channel"=w125:T7)  [unwired: 1 out]
    n143 = call <extravilib>:"Write.vi"("element"=w110) -> ("channel"=w124:T7)  [unwired: 1 out]
    n144 = call <extravilib>:"Write.vi"("element"=w111) -> ("channel"=w123:T7)  [unwired: 1 out]
  }
  n145 = while {
    tunnel: [w414] -> w21
    tunnel: w24 -> [w420]
    tunnel: w23 -> [w418]
    tunnel: [w411] -> w22
    tunnel: w12 -> [w410]
    tunnel: w7 -> [w409]
    tunnel: w6 -> [w408]
    tunnel: w5 -> [w407]
    tunnel: w4 -> [w406]
    tunnel: w3 -> [w405]
    tunnel: w2 -> [w404]
    tunnel: w1 -> [w402]
    stop <- w416 stop-if-true
    # "pre-cooling start time"
    # "ADR enabled"
    # "Desired temp"
    # "Low boundary"
    # "High boundary"
    # "TCP Named Service - Server Loop"
    n146 = call <extravilib>:"Read.vi"("channel"=w408) -> ("element"=w400:dbl)  [unwired: 1 in, 1 out]
    n147 = call <extravilib>:"Read.vi"("channel"=w402) -> ("element"=w403:T4)  [unwired: 1 in, 1 out]
    n148 = call <extravilib>:"Read.vi"("channel"=w404) -> ("element"=w391:dbl)  [unwired: 1 in, 1 out]
    n149 = call <extravilib>:"Read.vi"("channel"=w409) -> ("element"=w401:dbl)  [unwired: 1 in, 1 out]
    n150 = call <extravilib>:"Read.vi"("channel"=w407) -> ("element"=w399:dbl)  [unwired: 1 in, 1 out]
    n151 = call <extravilib>:"Read.vi"("channel"=w410) -> ("element"=w389:bool)  [unwired: 1 in, 1 out]
    n152 = call <extravilib>:"Read.vi"("channel"=w406) -> ("element"=w398:dbl)  [unwired: 1 in, 1 out]
    n153 = call <extravilib>:"Read.vi"("channel"=w405) -> ("element"=w397:bool)  [unwired: 1 in, 1 out]
    n154 = Unbundle By Name(w403) -> ("Start time"=w395:timestamp, "End time"=w394:timestamp, "duration"=w393:dbl[], "Price"=w392:dbl)  [unwired: 1 out]
    n155 = Subtract(x=w395, y=w391) -> (x-y=w396:timestamp)
    n156 = Bundle "System statuses"("element"=w389, "element"=w401, "element"=w400, "element"=w399, "element"=w398, "element"=w397, w396, "Start time"=w395, "End time"=w394, "duration"=w393, "Price"=w392, "element"=w391) -> (w390:T9)  [unwired: 1 in]
    n157 = TCP Wait On Listener(8:w418, 9:100 ("timeout ms (25000)"), 11:w420) -> (0:w419:errorcluster, 2:w412:string, 3:w411:refnum<k5>, 4:w417:refnum<k5>)  [unwired: 1 in, 1 out]
    n158 = case shown="No Error" w419 {
      selector: w419 -> [w429 w432]
      tunnel: [w427 w430] -> w414
      tunnel: w417 -> [w423 _]
      tunnel: w412 -> [_ _]
      tunnel: w390 -> [w421 _]
      frame No Error {
        # "The client is ready for data. Send a response string to the client."
        n159 = Flatten To String(anything=w421, prepend array or string size? (T)=TRUE, byte order (0:big-endian, network order)=T8."big-endian, network order") -> (data string=w422:string)  [unwired: 1 in, 2 out]
        n160 = TCP Write(connection ID=w423, data in=w422, error in (no error)=w429) -> (connection ID out=w426:refnum<k5>, error out=w428:errorcluster)  [unwired: 1 in, 1 out]
        n161 = TCP Close Connection(connection ID=w426, error in (no error)=w428) -> (error out=w427:errorcluster)  [unwired: 1 in, 1 out]
      }
      frame Error {
        # "Client did not send data. Ignore timeout error and keep waiting."
        n162 = Unbundle By Name(w432) -> ("code"=w431:i32)
        n163 = case shown="56" w431 {
          tunnel: w432 -> [w433 _]
          tunnel: [w433 w434] -> w430
          frame Default {
          }
          frame 56 {
            w434 = errorcluster {"status"=FALSE, "code"=0, "source"=""}  # No error
          }
        }
      }
    }
    n164 = Or(x=w414, y="Stop communication with PI") -> (x .or. y?=w416:bool)
  }
  n165 = while {
    tunnel: w12 -> [w464]
    shift-right: [w449] -> _
    shift-left: errorcluster {"status"=FALSE, "code"=0, "source"=""} ("error out") -> [w452]
    shift-right: ["Enable Logging 2"] -> _
    shift-left: _ -> [w453]
    tunnel: FALSE -> [w454]
    tunnel: w9 -> [w451]
    tunnel: w8 -> [w445]
    stop <- w449 stop-if-true
    w438 = 15.0 ("Time Target (s)")
    n166 = call <extravilib>:"Read.vi"("channel"=w451) -> ("element"=w450:dynamicdata)  [unwired: 1 in, 1 out]
    n167 = call <extravilib>:"Read.vi"("channel"=w464) -> ("element"=w448:bool)  [unwired: 1 in, 1 out]
    n168 = call <extravilib>:"Read.vi"("channel"=w445) -> ("element"=w442:dbl)  [unwired: 1 in, 1 out]
    n169 = Boolean To (0,1)(Boolean=w448) -> (0, 1=w447:i16)
    n170 = Build Array(w447) -> (w446:i16[])
    n171 = Not Equal?(x=w453, y=w454) -> (x != y?=w460:bool)
    n172 = Not And(1:"Append to Current File 2", 2:TRUE) -> (0:w456:bool)
    n173 = call-poly <vilib>:"Upsample.vi"("upsampling factor"=w442, "X"=w446) -> ("Upsampled Array"=w444:dbl[])  [unwired: 8 in, 1 out]
    n174 = call "Convert to Dynamic Data3"("Array"=w444) -> ("Dynamic Data Type"=w443:dynamicdata)  [unwired: 3 in]
    n175 = Merge Signals(w450, w443) -> (w441:dynamicdata)
    n176 = And(x=w460, y=w456) -> (x .and. y?=w459:bool)
    n177 = call "Elapsed Time"("Time Target (s)"=w438, "Auto Reset"=TRUE) -> ("Elapsed Time (s)"=w439:dbl)  [unwired: 10 in, 7 out]
    n178 = Greater Or Equal?(x=w439, y=w438) -> (x >= y?=w437:bool)
    n179 = xnode "Set Dynamic Data Attributes"("Signals In"=w441) -> ("Signals Out"=w435:dynamicdata)  [unwired: 3 in, 1 out]
    n180 = case shown="True" w437 {
      tunnel: [_ w465] -> w436
      tunnel: w435 -> [_ w465]
      frame False {
      }
      frame True {
      }
    }
    n181 = call "Write To Measurement File"("Signals"=w436, "Enable"="Enable Logging 2", "new_file"=w459, "error in (no error)"=w452, "Filename"="Path to log file 2") -> ("Saving Data"=→"Saving/Logging Data 2":bool, "error out"=w449:errorcluster)  [unwired: 12 in, 1 out]
    n182 = Wait (ms)(milliseconds to wait=u32 1000) -> ()  [unwired: 1 out]
  }
  n183 = TCP Close Connection(connection ID=w22, error in (no error)=w21) -> (error out=w20:errorcluster)  [unwired: 1 in, 1 out]
  n184 = call <vilib>:"Simple Error Handler.vi"("error in (no error)"=w20) -> ()  [unwired: 4 in, 5 out]
